vi "Subscribe.vi"(8 "error in":errorcluster, 9 "Message":refnum<class "Message.lvclass">, 10 "Enqueuer":refnum<class "Message Enqueuer.lvclass">, 11 "MVC Subscription in":refnum<class "MVC Subscription.lvclass">) -> (0 "error out":errorcluster, 3 "MVC Subscription out":refnum<class "MVC Subscription.lvclass">)   [LabVIEW 2014, in "MVC Subscription.lvlib" / "MVC Subscription.lvclass"]
uses:
  MVC Subscription.lvclass
  <vilib>/ActorFramework/Message Enqueuer/Message Enqueuer.lvclass
  <vilib>/ActorFramework/Message/Message.lvclass
  Cluster - Individual Subscription.ctl
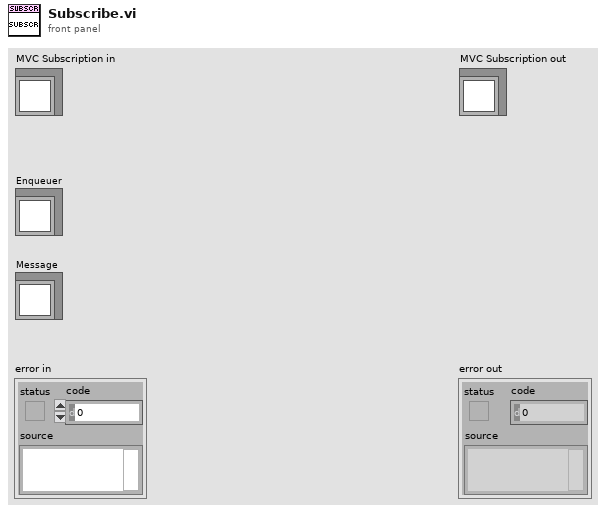
[diagram p1: front panel]
types:
  T1 = typedef "MVC Subscription.lvlib/MVC Subscription.lvclass/Cluster - Individual Subscription.ctl" = cluster{"Enqueuer":refnum<class "Message Enqueuer.lvclass">, "Message":refnum<class "Message.lvclass">}
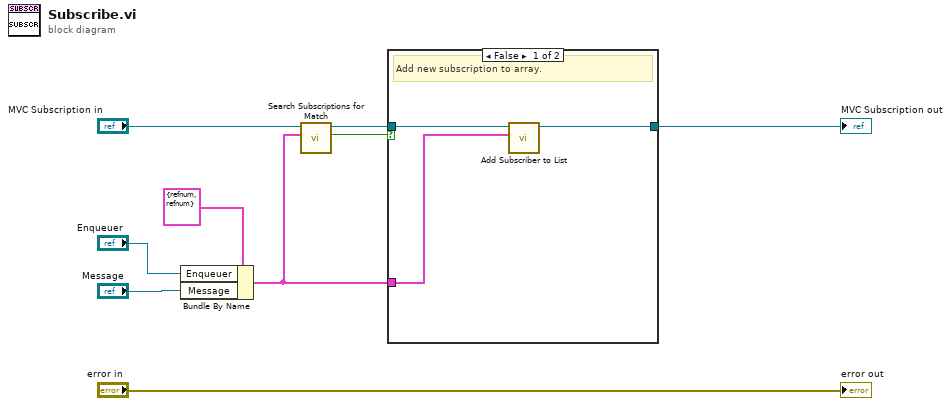
[diagram p0: block diagram]
diagram:
  n1 = Bundle By Name(cluster=T1 {"Enqueuer"=refnum, "Message"=refnum} ("Subscription"), "Enqueuer"="Enqueuer", "Message"="Message") -> (w1:T1)
  n2 = call "Search Subscriptions for Match.vi"("Subscription"=w1, "MVC Subscription in"="MVC Subscription in") -> ("Found"=w2:bool, "MVC Subscription out"=w3:refnum<class "MVC Subscription.lvclass">)  [unwired: 7 in, 1 out]
  n3 = case shown="False" w2 {
    tunnel: [w12 w13] -> w4
    tunnel: w3 -> [w11 w13]
    tunnel: w1 -> [w10 _]
    frame False {
      # "Add new subscription to array."
      n4 = call "Add Subscriber to List.vi"("Subscription"=w10, "MVC Subscription in"=w11) -> ("MVC Subscription out"=w12:refnum<class "MVC Subscription.lvclass">)  [unwired: 9 in]
    }
    frame True {
      # "Subscription already present. Do nothing."
    }
  }
  "MVC Subscription out" <- w4
  "error out" <- "error in"
